vi "Complex FFT.vi"(9 "FFT size":i32=-1, 10 "shift?":bool, 11 "X":cdb[](array[numeric])) -> (0 "error":i32, 3 "FFT {X}":cdb[](array[numeric]))   [LabVIEW 2017, in "NI_AALPro.lvlib"]
doc: "Computes the fast Fourier transform (FFT) of the input sequence <B>X</B>. Wire data to the <B>X</B> input to determine the polymorphic instance to use or manually select the instance."
uses:
  NI_AALPro.lvlib
  lvanlys.dll
panel:
  # "Complex FFT"
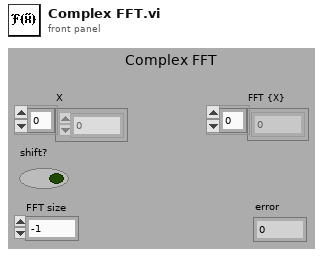
[diagram p1: front panel]
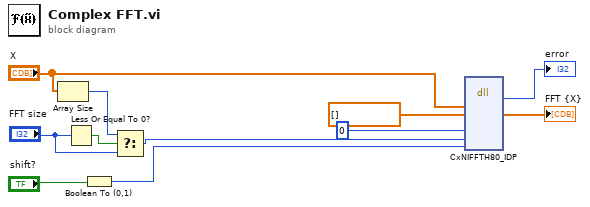
[diagram p0: block diagram]
diagram:
  n1 = Array Size(array="X") -> (size(s)=w10:i32)
  n2 = Less Or Equal To 0?(x="FFT size") -> (x <= 0?=w11:bool)
  n3 = Boolean To (0,1)(Boolean="shift?") -> (0, 1=w5:i16)
  n4 = Select(t=w10, s=w11, f="FFT size") -> (s? t:f=w7:i32)
  n5 = dll-call lib="C:/Program Files/National Instruments/LabVIEW 2017/resource/lvanlys.*" fn="CxNIFFTH80_IDP"("xH"="X", "yH"=cdb[] [] ("FFT {X}"), "org"=0, "fftSize"=w7, "shift"=w5) -> ("return type"=→"error":i32, "yH"=→"FFT {X}":cdb[])  [unwired: 9 in, 2 out]
